vi "FPGA Main.vi"   [LabVIEW 2019]
uses:
  targets/Bank List.ctl
  api/Bank/Bank Type.ctl
  <vilib>/Platform/TimedLoop/XDataNode/timing_clust.ctl
  <vilib>/Platform/TimedLoop/XDataNode/nitl_modes.ctl
  <vilib>/Platform/TimedLoop/XDataNode/wakeup.ctl
  <vilib>/rvi/Emulation/niFpgaSctlEmulationGetInTimedLoop.vi
  <vilib>/rvi/Emulation/niFpgaEmulationReportErrorSimple.vi
  <vilib>/rvi/Emulation/niFpgaGetClockAttributes.vi
  <vilib>/rvi/Emulation/niFpgaCriticalErrorInLSC.vi
  <vilib>/platform/TimedLoop/XDataNode/XDataNode.xnode
  <vilib>/Platform/TimedLoop/XDataNode/XDNodeRunTimeDep.lvlib
  api/Bank/Bank.lvclass
types:
  T1 = typedef "Bank.lvclass/Bank Type.ctl" = enum16{"None", "Discrete Acquisition", "Discrete Generation", "PWM Acquisition", "PWM Generation"}
  T2 = typedef "Bank.lvclass/Bank List.ctl" = enum16{"Connector 0/Bank 0", "Connector 0/Bank 1", "Connector 0/Bank 2", "Connector 0/Bank 3", "Connector 1/Bank 0", "Connector 1/Bank 1", "Connector 1/Bank 2", "Connector 1/Bank 3", "Connector 2/Bank 0", "Connector 2/Bank 1", "Connector 2/Bank 2", "Connector 2/Bank 3", "Connector 3/Bank 0", "Connector 3/Bank 1", "Connector 3/Bank 2", "Connector 3/Bank 3"}
  T3 = typedef "XDNodeRunTimeDep.lvlib/timing_clust.ctl" = cluster{"Expected End [f-1]":u64, "Actual End [f-1]":u64, "Finished Late? [f-1]":bool, "Expected End [i-1]":u64, "Actual End [i-1]":u64, "Finished Late? [i-1]":bool, "Expected Start [i]":u64, "Actual Start [i]":u64, "Expected Start [f]":u64, "Actual Start [f]":u64, "Source Name":string, "Structure Name":string, "Period":i64, "Deadline":i64, "Offset":i64, "Start":i64, "Priority":i32, "Timeout":i32, "Mode":T4, "Wakeup Reason":T5, "Error":errorcluster, "Source Type":string, "Secondary Source Type":string, "Global End Time":u64, "Global Start Time":u64, "Frame Duration":u64, "Iteration Duration":u64, "Assigned CPU":i32, "I/O Scan Engine Mode":u32}
  T4 = typedef "XDNodeRunTimeDep.lvlib/nitl_modes.ctl" = enum32{"No Change", "Process missed periods, maintain original phase", "Discard missed periods, maintain original phase", "Process missed periods, ignore original phase", "Discard missed periods, ignore original phase"}
  T5 = typedef "XDNodeRunTimeDep.lvlib/wakeup.ctl" = enum32{"Normal", "Aborted", "Asynchronous wakeup", "Timing source error", "Timed loop error", "Timeout"}
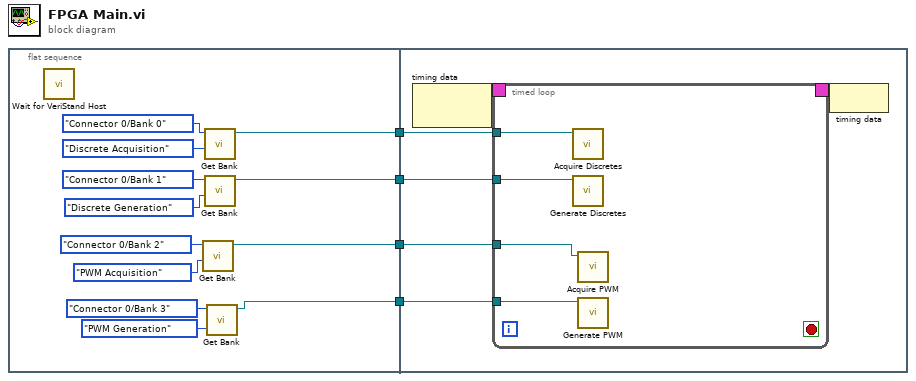
[diagram p0: block diagram]
diagram:
  n1 = flat-sequence {
    tunnel: [w14] -> w4
    tunnel: [w13] -> w3
    tunnel: [w8] -> w2
    tunnel: [w5] -> w1
    tunnel: w4 -> [w20]
    tunnel: w3 -> [w19]
    tunnel: w2 -> [w18]
    tunnel: w1 -> [w17]
    frame #0 {
      n2 = call "Wait for VeriStand Host.vi"() -> ()  [unwired: 12 in]
      n3 = call "Get Bank.vi"("Bank Type"=Bank_Type."PWM Acquisition", 11:Bank_List."Connector 0/Bank 2") -> ("Bank out"=w8:refnum<class "Bank.lvclass">)  [unwired: 9 in]
      n4 = call "Get Bank.vi"("Bank Type"=Bank_Type."Discrete Acquisition", 11:Bank_List."Connector 0/Bank 0") -> ("Bank out"=w13:refnum<class "Bank.lvclass">)  [unwired: 9 in]
      n5 = call "Get Bank.vi"("Bank Type"=Bank_Type."Discrete Generation", 11:Bank_List."Connector 0/Bank 1") -> ("Bank out"=w14:refnum<class "Bank.lvclass">)  [unwired: 9 in]
      n6 = call "Get Bank.vi"("Bank Type"=Bank_Type."PWM Generation", 11:Bank_List."Connector 0/Bank 3") -> ("Bank out"=w5:refnum<class "Bank.lvclass">)  [unwired: 9 in]
    }
    frame #1 {
      n7 = node-c288() -> (w22:T3)  [unwired: 1 in]
      n8 = timed-loop {
        timing: w22 -> [_]
        timing-out: [_] -> w21
        tunnel: w20 -> [w26]
        tunnel: w19 -> [w25]
        tunnel: w18 -> [w24]
        tunnel: w17 -> [w23]
        stop <- _ stop-if-true
        n9 = call "Acquire Discretes.vi"("Bank in"=w25) -> ()  [unwired: 9 in, 2 out]
        n10 = call "Generate Discretes.vi"("Bank in"=w26) -> ()  [unwired: 10 in, 1 out]
        n11 = call "Acquire PWM.vi"("Bank in"=w24) -> ()  [unwired: 9 in, 2 out]
        n12 = call "Generate PWM.vi"("Bank in"=w23) -> ()  [unwired: 9 in, 2 out]
      }
      n13 = node-c288(w21) -> ()
    }
  }
